vi "Remove Component.vi"(8 "error in (no error)":errorcluster, 10 "Item":refnum<class "Item.lvclass">, 11 "Blueprint in":refnum<class "Blueprint.lvclass">) -> (0 "error out":errorcluster, 3 "Blueprint out":refnum<class "Blueprint.lvclass">)   [LabVIEW 2020, in "Blueprint.lvclass"]
uses:
  Blueprint.lvclass
  Item/Item.lvclass
  Blueprint.lvclass/Blueprint.ctl
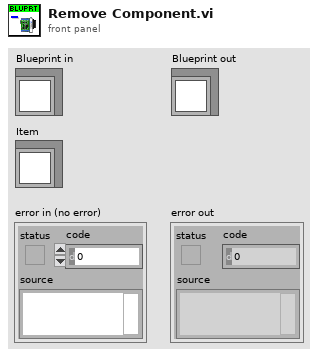
[diagram p1: front panel]
types:
  T1 = typedef "Blueprint.lvclass/Ref Data.ctl" = cluster{"Ingredients":T2[], "Workstation":refnum<class "Workstation.lvclass">, "Craft Time":dbl, "Name":string}
  T2 = typedef "Item.lvclass/Ingredient.ctl" = cluster{"Item":refnum<class "Item.lvclass">, "Qty":dbl}
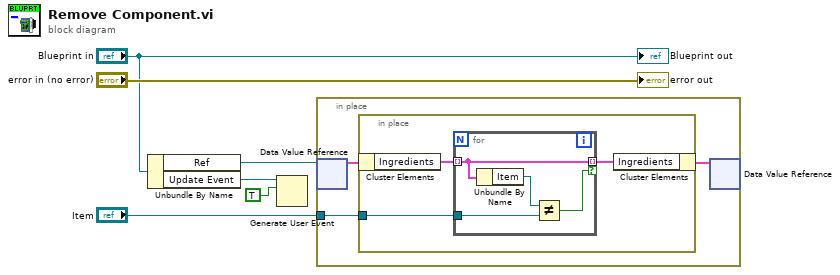
[diagram p0: block diagram]
diagram:
  n1 = Unbundle By Name("Blueprint in") -> ("Ref"=w5:refnum<data-value>, "Update Event"=w2:refnum<user-event>)
  n2 = Generate User Event(user event=w2, event data cluster=TRUE ("event data")) -> ()  [unwired: 2 in, 2 out]
  n3 = in-place {
    in-place-border: "Item" -> [w7]
    n4 = in-place-dvr #1(w5) -> (w9:T1)  [unwired: 1 out]
    n5 = in-place {
      in-place-border: w7 -> [w12]
      n6 = in-place-cluster #2(w9) -> ("Ingredients"=w11:T2[])
      n7 = for {
        tunnel: w12 -> [w16]
        tunnel: w11 -> [w14] mode=indexing
        tunnel: [w14] -> w10 mode=indexing if=w13
        n8 = Unbundle By Name(w14) -> ("Item"=w15:refnum<class "Item.lvclass">)
        n9 = Not Equal?(x=w15, y=w16) -> (x != y?=w13:bool)
      }
      n10 = in-place-cluster #2("Ingredients"=w10) -> (w8:T1)
    }
    n11 = in-place-dvr #1(w8) -> ()  [unwired: 2 out]
  }
  "error out" <- "error in (no error)"
  "Blueprint out" <- "Blueprint in"
